vi "IDE_Folder_Example.vi"() -> ()   [LabVIEW 2020]
uses:
  Subs/ColorText/Code.xctl
  Subs/Console XCtrl/Console_Xctrl.xctl
  Subs/Server XCtrl/Server.xctl
panel:
  in  "New":bool
  in  "Base Path":path
  in  "Tree":string(tree)
  in  "Clean":bool
  in  "PC Save":bool
  in  "Files":bool
  in  "Server":bool
  in  "Help":bool
  in  "Server":path(xcontrol)=path "/Users/crogers/GitHub/Summer2020/LabVIEWCode/Servers/Jens.vi"
  out "REPL":string(xcontrol)
  in  "Clear":bool
  in  "Save":bool
  in  "Stop":bool
  in  "Run":bool
  in  "Name":string="code.py"
  in  "Code":string(xcontrol)="import os\n\nfor i in range(10):\n     print(i)\n"
  # "¨Processor"
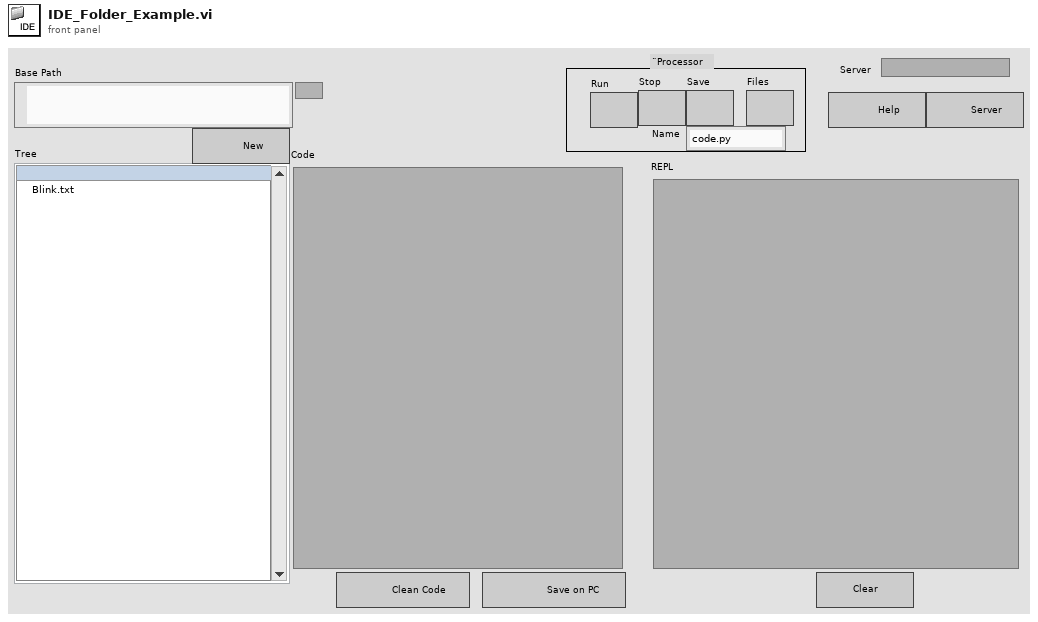
[diagram p1: front panel]
types:
  T1 = cluster{"Quote":u32, "Comment":u32, "Python":u32, "Text":u32, "Triple Quote":u32, "function":u32, "Line numbers":u32, "REPL Err":u32, "REPL Text":u32, "Text Bkgd":u32, "REPL Bkgd":u32}
  T2 = enum8{"Enabled", "Disabled", "Disabled and Grayed Out"}
  T3 = typedef "eventvkey.ctl" = enum16{"ASCII", "Enter", "Return", "Shift", "Ctrl", "Alt", "Cmd", "Opt", "Caps", "NumLock", "Clear", "Break", "Up", "Down", "Left", "Right", "Insert", "Delete", "Home", "End", "PageUp", "PageDown", "Escape", "Help", "Pause", "ScrollLock", "F1", "F2", "F3", "F4", "F5", "F6", "F7", "F8", "F9", "F10", "F11", "F12", "F13", "F14", "F15", "F16", "F17", "F18", "F19", "F20", "F21", "F22", "F23", "F24", "Play", "VolumeUp", "VolumeDown", "Mute", "Two Byte Char"}
  T4 = cluster{"Shift":bool, "Ctrl":bool, "Alt":bool, "Cmd":bool, "Opt":bool}
  T5 = cluster{"Char":i16, "VKey":T3, "PlatMods":cluster{"Shift":bool, "Ctrl":bool, "Alt":bool, "Cmd":bool, "Opt":bool}}
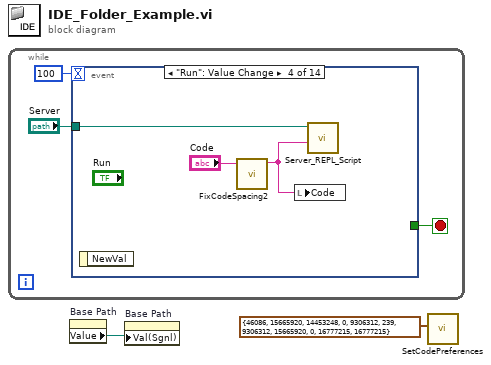
[diagram p0: block diagram]
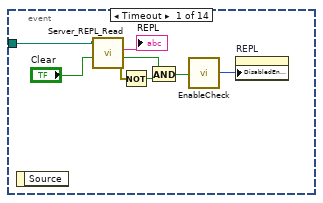
[diagram p2: hidden frame]
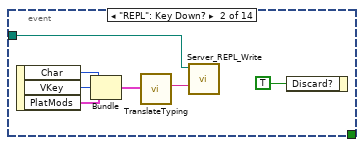
[diagram p3: hidden frame]
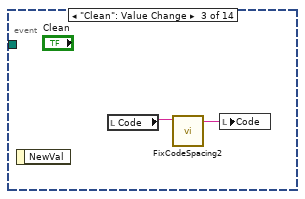
[diagram p4: hidden frame]
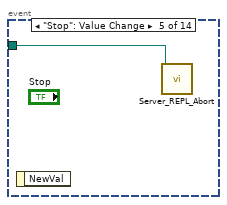
[diagram p5: hidden frame]
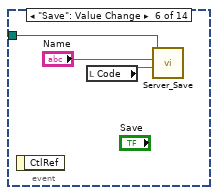
[diagram p6: hidden frame]
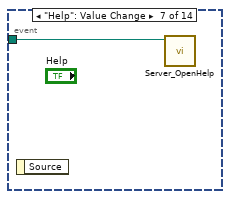
[diagram p7: hidden frame]
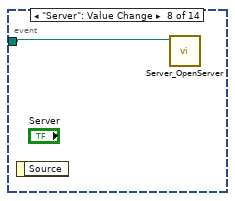
[diagram p8: hidden frame]
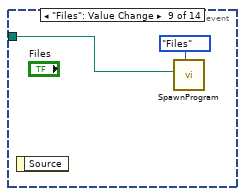
[diagram p9: hidden frame]
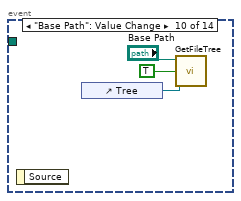
[diagram p10: hidden frame]
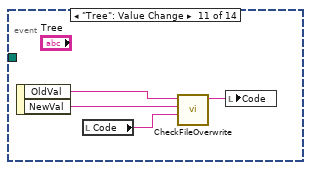
[diagram p11: hidden frame]
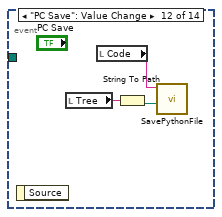
[diagram p12: hidden frame]
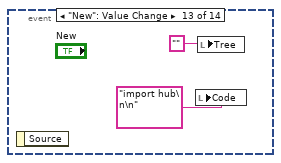
[diagram p13: hidden frame]
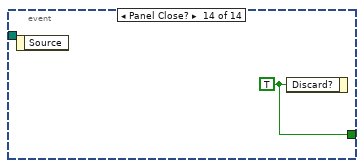
[diagram p14: hidden frame]
diagram:
  n1 = while {
    stop <- w4 stop-if-true
    n2 = event shown="[3] \"Run\": Value Change" {
      selector: _ -> [_ _ _ _ _ _ _ _ _ _ _ _ _ _]
      dyn-events: _ -> [_ _ _ _ _ _ _ _ _ _ _ _ _ _]
      timeout: 100 -> [_ _ _ _ _ _ _ _ _ _ _ _ _ _]
      tunnel: [_ _ _ _ _ _ _ _ _ _ _ _ _ w46] -> w4
      tunnel: "Server" -> [w12 w14 _ w24 w26 w27 w30 w31 w33 _ _ _ _ _]
      event Timeout {
        n3 = event-data() -> ()  [unwired: 1 in, 1 out]
        n4 = call "Server_REPL_Read.vi"("Clear"="Clear", "Server"=w12) -> ("error out"=w8:errorcluster, "Running?"=w9:bool, "REPL"=→"REPL":string)  [unwired: 7 in]
        n5 = Not(x=w8) -> (.not. x?=w7:bool)
        n6 = And(x=w9, y=w7) -> (x .and. y?=w6:bool)
        n7 = call "EnableCheck.vi"("Enable?"=w6) -> ("Enum"=w13:T2)
        n8 = property on="REPL" class="Console_Xctrl (strict)"("DisabledEnum"=w13) -> ()  [unwired: 2 in, 2 out]
      }
      event "REPL": Key Down? {
        n9 = event-data() -> ("Char"=w19:i16, "VKey"=w18:T3, "PlatMods"=w16:T4)  [unwired: 1 in]
        n10 = Bundle("Char"=w19, "VKey"=w18, "PlatMods"=w16) -> (w20:T5)  [unwired: 1 in]
        n11 = call "TranslateTyping.vi"("Cluster"=w20) -> ("key"=w15:string)  [unwired: 10 in]
        n12 = call "Server_REPL_Write.vi"("Code"=w15, "Server"=w14) -> ()  [unwired: 9 in, 1 out]
        n13 = event-data("Discard?"=TRUE) -> ()  [unwired: 1 in, 1 out]
      }
      event "Clean": Value Change {
        n14 = event-data() -> ()  [unwired: 1 in, 1 out]
        n15 = local read "Code"() -> (w21:string)
        n16 = call "FixCodeSpacing2.vi"("Code"=w21) -> ("Cleaned"=w22:string)  [unwired: 10 in]
        n17 = local write "Code"(w22) -> ()
      }
      event "Run": Value Change {
        n18 = event-data() -> ()  [unwired: 1 in, 1 out]
        n19 = call "FixCodeSpacing2.vi"("Code"="Code") -> ("Cleaned"=w23:string)  [unwired: 10 in]
        n20 = local write "Code"(w23) -> ()
        n21 = call "Server_REPL_Script.vi"("Code"=w23, "Server"=w24) -> ()  [unwired: 9 in, 1 out]
      }
      event "Stop": Value Change {
        n22 = event-data() -> ()  [unwired: 1 in, 1 out]
        n23 = call "Server_REPL_Abort.vi"("Server"=w26) -> ()  [unwired: 10 in, 1 out]
      }
      event "Save": Value Change {
        n24 = event-data() -> ()  [unwired: 1 in, 1 out]
        n25 = local read "Code"() -> (w29:string)
        n26 = call "Server_Save.vi"("Code"=w29, "Name"="Name", "Server"=w27) -> ()  [unwired: 8 in, 1 out]
      }
      event "Help": Value Change {
        n27 = event-data() -> ()  [unwired: 1 in, 1 out]
        n28 = call "Server_OpenHelp.vi"("Server"=w30) -> ()  [unwired: 10 in, 1 out]
      }
      event "Server": Value Change {
        n29 = event-data() -> ()  [unwired: 1 in, 1 out]
        n30 = call "Server_OpenServer.vi"("Server"=w31) -> ()  [unwired: 10 in, 1 out]
      }
      event "Files": Value Change {
        n31 = event-data() -> ()  [unwired: 1 in, 1 out]
        n32 = call "SpawnProgram.vi"("Server"=w33, "Dialog"=enum16{"Help", "Files"}."Files") -> ()  [unwired: 10 in]
      }
      event "Base Path": Value Change {
        n33 = event-data() -> ()  [unwired: 1 in, 1 out]
        n34 = control-ref of="Tree"() -> (w36:refnum<vi>)
        n35 = call "GetFileTree.vi"("Tree"=w36, "Open?"=TRUE, "Base Path"="Base Path") -> ()  [unwired: 9 in]
      }
      event "Tree": Value Change {
        n36 = event-data() -> ("OldVal"=w40:string, "NewVal"=w37:string)  [unwired: 1 in]
        n37 = local read "Code"() -> (w38:string)
        n38 = call "CheckFileOverwrite.vi"("Current Code"=w38, "New Value"=w37, "Old Value"=w40) -> ("Code out"=w39:string)  [unwired: 8 in]
        n39 = local write "Code"(w39) -> ()
      }
      event "PC Save": Value Change {
        n40 = event-data() -> ()  [unwired: 1 in, 1 out]
        n41 = local read "Tree"() -> (w43:string)
        n42 = local read "Code"() -> (w42:string)
        n43 = String To Path(string=w43) -> (path=w41:path)
        n44 = call "SavePythonFile.vi"("path"=w41, "Code"=w42) -> ()  [unwired: 10 in]
      }
      event "New": Value Change {
        n45 = event-data() -> ()  [unwired: 1 in, 1 out]
        n46 = local write "Code"("import hub\n\n") -> ()
        n47 = local write "Tree"("") -> ()
      }
      event Panel Close? {
        w46 = TRUE ("Discard?")
        n48 = event-data() -> ()  [unwired: 1 in, 1 out]
        n49 = event-data("Discard?"=w46) -> ()  [unwired: 1 in, 1 out]
      }
    }
  }
  n50 = property on="Base Path" class="Path"() -> ("Value"=w1:path)  [unwired: 2 in, 2 out]
  n51 = property on="Base Path" class="Path"("Val(Sgnl)"=w1) -> ()  [unwired: 2 in, 2 out]
  n52 = call "SetCodePreferences.vi"("Color choices"=T1 {"Quote"=46086, "Comment"=15665920, "Python"=14453248, "Text"=0, "Triple Quote"=9306312, "function"=239, "Line numbers"=9306312, "REPL Err"=15665920, "REPL Text"=0, "Text Bkgd"=16777215, "REPL Bkgd"=16777215}) -> ()  [unwired: 11 in]
